vi "LoadCompiledString.vi"(0 "Compiled String":string="#DopplerCooling\r\n0.9 10100000 00000000 00000000\r\n\r\n#Pump\r\n0.3 01000000 00000000 00000000\r\n\r\n#Pulsed\r\n0.2 00100000 00000000 00000000\r\n0.4 00000100 00000000 00000000\r\n0.2 00000000 10000000 00000000\r\n0.2 01000000 00000000 01000000\n") -> (1 "Durations":dbl[](array[numeric]), 2 "States":string[](array[string]), 3 "ChapterNames":string[](array[string]), 4 "ChapterPositions":u32[](array[numeric]))   [LabVIEW 2014]
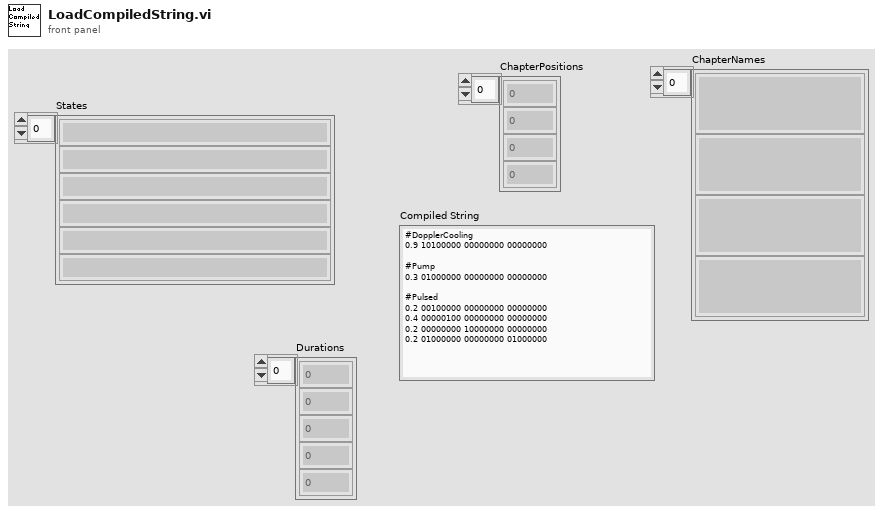
[diagram p1: front panel]
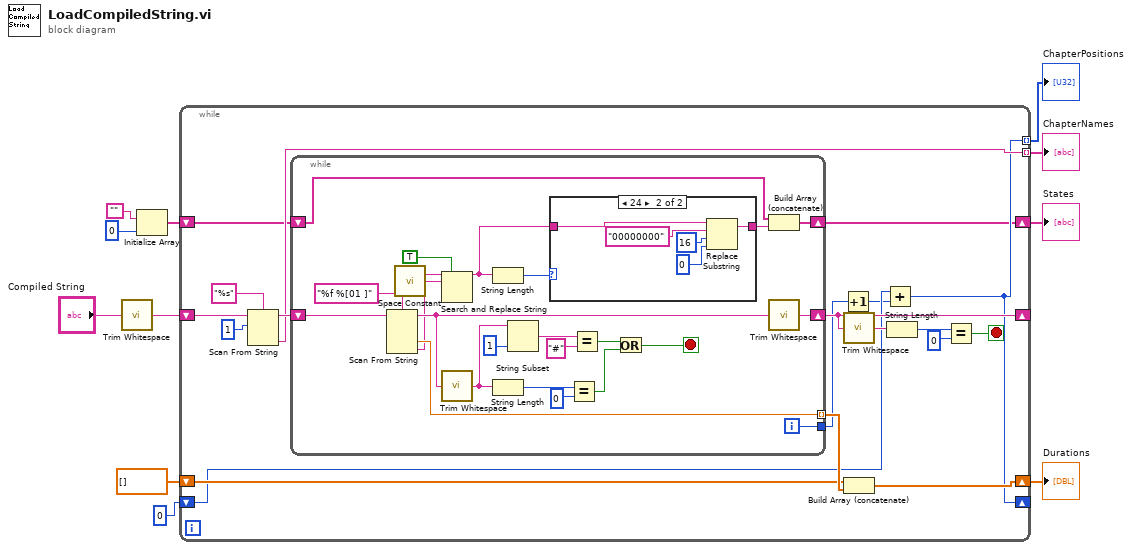
[diagram p0: block diagram]
diagram:
  n1 = call <vilib>:"Trim Whitespace.vi"("string"="Compiled String") -> ("trimmed string"=w1:string)  [unwired: 1 in]
  n2 = Initialize Array("", 0 ("dimension size")) -> (w6:string[])
  n3 = while {
    shift-right: [w27] -> w11
    shift-left: dbl[] [] -> [w25]
    tunnel: [w24] -> w9 mode=indexing
    shift-right: [w19] -> _
    shift-left: w1 -> [w23]
    shift-right: [w14] -> _
    shift-left: u32 0 ("initial scan location") -> [w16]
    tunnel: [w14] -> w7 mode=indexing
    shift-right: [w12] -> w3
    shift-left: w6 -> [w13]
    stop <- w20 stop-if-true
    n4 = Scan From String(format string="%s", input string=w23, initial scan location=u32 1) -> (remaining string=w29:string, output 1=w24:string)  [unwired: 2 in, 2 out]
    n5 = while {
      tunnel: [w51] -> w26 mode=indexing
      shift-right: [w48] -> w19
      shift-left: w29 -> [w53]
      tunnel: [w39] -> w17
      shift-right: [w37] -> w12
      shift-left: w13 -> [w38]
      i -> [w39]
      stop <- w42 stop-if-true
      n6 = Scan From String(format string="%f %[01 ]", input string=w53) -> (remaining string=w41:string, output 1=w51:dbl, output 2=w36:string)  [unwired: 4 in, 2 out]
      n7 = call <vilib>:"Space Constant.vi"() -> ("String"=w35:string)
      n8 = Search and Replace String(replace all?=TRUE ("replace all? (F)"), input string=w36, search string=w35) -> (result string=w32:string)  [unwired: 5 in, 3 out]
      n9 = call <vilib>:"Trim Whitespace.vi"("string"=w41) -> ("trimmed string"=w40:string)  [unwired: 1 in]
      n10 = String Length(string=w32) -> (length=w33:i32)
      n11 = String Length(string=w40) -> (length=w50:i32)
      n12 = String Subset(string=w40, length (rest)=1 ("line index")) -> (substring=w46:string)  [unwired: 1 in]
      n13 = case shown="24" w33 {
        tunnel: [w54 w56] -> w31
        tunnel: w32 -> [w54 w55]
        frame 32, Default {
        }
        frame 24 {
          n14 = Replace Substring(2:0 ("length (len. of substring)"), 3:16 ("offset (0)"), 4:"00000000" ("substring (\"\")"), 5:w55) -> (1:w56:string)  [unwired: 1 out]
        }
      }
      n15 = Equal?(x=w50, y=0) -> (x = y?=w43:bool)
      n16 = Equal?(x=w46, y="#") -> (x = y?=w44:bool)
      n17 = Or(x=w44, y=w43) -> (x .or. y?=w42:bool)
      n18 = Build Array (concatenate)(w38, w31) -> (w37:string[])
      n19 = call <vilib>:"Trim Whitespace.vi"("string"=w41) -> ("trimmed string"=w48:string)  [unwired: 1 in]
    }
    n20 = Increment(x=w17) -> (x+1=w15:i32)
    n21 = call <vilib>:"Trim Whitespace.vi"("string"=w19) -> ("trimmed string"=w18:string)  [unwired: 1 in]
    n22 = Build Array (concatenate)(w25, w26) -> (w27:dbl[])
    n23 = Add(x=w16, y=w15) -> (x+y=w14:u32)
    n24 = String Length(string=w18) -> (length=w22:i32)
    n25 = Equal?(x=w22, y=0) -> (x = y?=w20:bool)
  }
  "Durations" <- w11
  "ChapterNames" <- w9
  "ChapterPositions" <- w7
  "States" <- w3
